vi "PID play.vi"() -> ()   [LabVIEW 2009]
panel:
  out "output cluster":cluster{"setpoint":dbl, "output":dbl}
  in  "instantaneous":dbl(slide) scale=-10.0..10.0
  in  "multiplier":dbl
  in  "parameters":cluster{"P":dbl, "I":dbl, "D":dbl}
  in  "setpoint":dbl(slide) scale=0.0..100.0
  in  "response time (ms)":u32=20
  in  "STOP":bool
  in  "slope":dbl(slide) scale=-50.0..50.0
  out "Waveform Chart":cluster{dbl, "P":dbl}(graph)
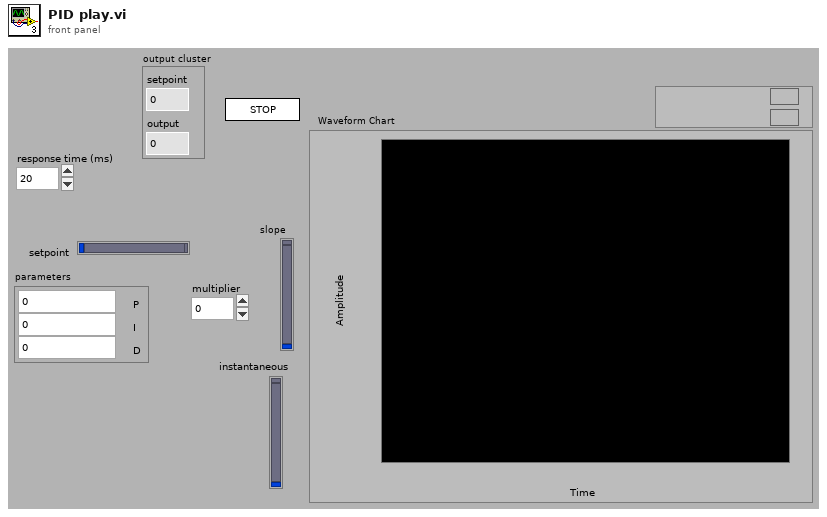
[diagram p1: front panel]
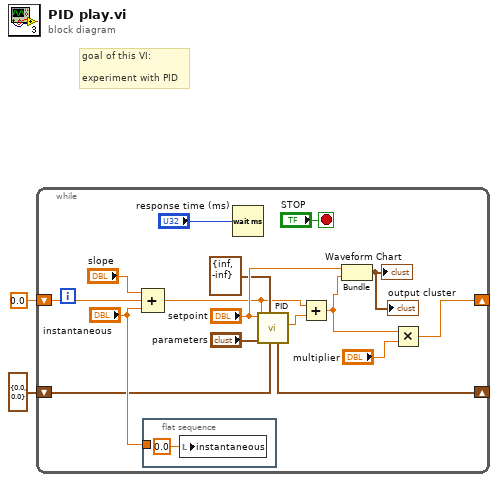
[diagram p0: block diagram]
diagram:
  # "goal of this VI:\n\nexperiment with PID"
  n1 = while {
    shift-right: [w12] -> _
    shift-left: 0.0 -> [w10]
    shift-right: [w7] -> _
    shift-left: cluster{"error":dbl, "integral":dbl} {"error"=0.0, "integral"=0.0} ("previous (out)") -> [w8]
    stop <- "STOP" stop-if-true
    n2 = Compound Arithmetic op=ADD("slope", w10, "instantaneous") -> (w4:dbl)
    n3 = flat-sequence {
      tunnel: "instantaneous" -> [_]
      frame #0 {
        n4 = local write "instantaneous"(0.0 ("instantaneous")) -> ()
      }
    }
    n5 = Wait (ms)(milliseconds to wait="response time (ms)") -> ()  [unwired: 1 out]
    n6 = call "PID.vi"("previous (in)"=w8, "range"=cluster{"max":dbl, "min":dbl} {"max"=inf, "min"=-inf}, "coeffecients"="parameters", "process variable"=w4, "setpoint"="setpoint") -> ("output"=w5:dbl, "previous (out)"=w7:cluster{"error":dbl, "integral":dbl})  [unwired: 5 in]
    n7 = Add(x=w4, y=w5) -> (x+y=w3:dbl)
    n8 = Bundle("setpoint"="setpoint", w3) -> (→"Waveform Chart" →"output cluster":cluster{"setpoint":dbl, dbl})  [unwired: 1 in]
    n9 = Multiply(x=w3, y="multiplier") -> (x*y=w12:dbl)
  }
